vi "Periodic Tasks.vi"(8 "error in":errorcluster) -> ()   [LabVIEW 2019]
doc: "This VI runs in parallel to other tasks. It can contain as many user-defined periodic loops as you need. These can carry out PID or other sorts of timed response."
uses:
  <vilib>/Rock Robotics/WPI/ThirdParty/Phoenix-LabVIEW/Motor Controller/Controls/CTRE_Phoenix_MotorControl_ControlMode.ctl
  <vilib>/Rock Robotics/WPI/Solenoid/WPI_SolenoidValue.ctl
  Ball Routine.ctl
  TurretMode.ctl
  LabVIEW_is_Under_Control.lib/Util/Toggle/Change Detect.vi
  LabVIEW_is_Under_Control.lib/Util/Toggle/Change Detect Boolean.vi
  MotorsGlobal.vi
  <vilib>/Rock Robotics/WPI/Solenoid/WPI_SolenoidSetEnum.vi
  <vilib>/Rock Robotics/Network Tables/NT Read Number.vi
  JoysticksGlobal.vi
  <vilib>/Rock Robotics/WPI/Utilities/WPI_GetSetVariantRefNum.vi
  <vilib>/Rock Robotics/Network Tables/NT Write Number.vi
panel:
  out "Encoder Out":dbl
  in  "PIDs Tab":T1(tab)
  out "Current":dbl
  out "Motor Temperature":u8
  out "Current 2":dbl
  out "Motor Temperature 2":u8
  out "Current 3":dbl
  out "Motor Temperature 3":u8
  out "Current 4":dbl
  out "Motor Temperature 4":u8
  out "LimelightX":dbl
  out "Turret PID":cluster{"Setpoint":dbl, "Process variable":dbl}(graph)
  in  "Camera Angle":dbl=7.0
  out "Distancia do Goal":dbl
  in  "Inner Goal Height":dbl=2.49
  in  "Camera Height":dbl=0.185
  in  "Minimum command":dbl=0.031
  out "Turret Out":dbl
  in  "TAGains":T2={"proportional gain (Kc)"=1.0, "integral time (Ti, min)"=0.01, "derivative time (Td, min)"=0.0} {"derivative time (Td, min)" format="%.3f"; "integral time (Ti, min)" format="%.3f"; "proportional gain (Kc)" format="%.3f"}
  in  "TADisable Range":dbl
  in  "TAIntegral Range":dbl=10000.0
  in  "TASetpoint":dbl
  in  "TARange":cluster{"output high":dbl, "output low":dbl}={"output high"=0.6, "output low"=-0.6} {"output low" format="%.2f"; "output high" format="%.2f"}
  in  "kF":dbl=0.031
  out "Shooter PID":cluster{"Setpoint":dbl, "Process variable":dbl}(graph)
  in  "EnableFWPID":bool
  out "Variable":dbl
  in  "FWGains":T2={"proportional gain (Kc)"=1.0, "integral time (Ti, min)"=0.01, "derivative time (Td, min)"=0.0} {"derivative time (Td, min)" format="%.3f"; "integral time (Ti, min)" format="%.3f"; "proportional gain (Kc)" format="%.3f"}
  in  "FWRange":cluster{"output high":dbl, "output low":dbl}={"output high"=0.6, "output low"=-0.6} {"output low" format="%.2f"; "output high" format="%.2f"}
  in  "FWIntegral Range":dbl=10000.0
  in  "FWSetpoint":dbl
  in  "FWDisable Range":dbl
  # "System Tester"
  # "ID-1"
  # "ID-3"
  # "ID-2"
  # "ID-4"
  # "Distance Meter"
  # "All in cm"
  # "Turret Angle PID"
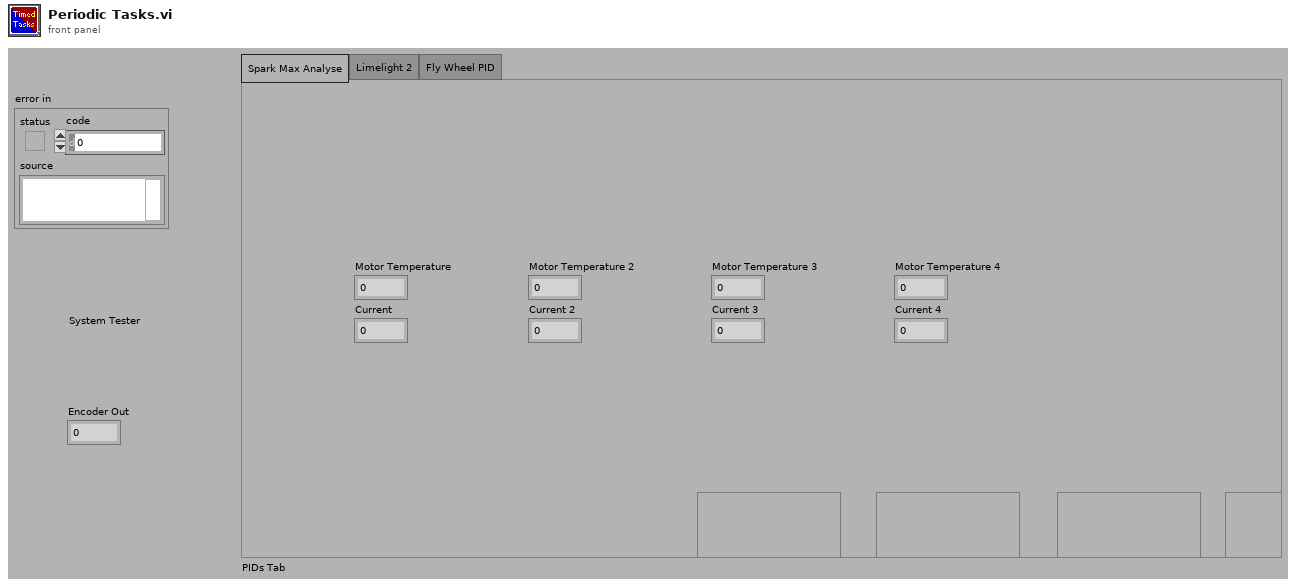
[diagram p1: front panel]
types:
  T1 = enum32{"Spark Max Analyse", "Limelight 2", "Fly Wheel PID"}
  T2 = cluster{"proportional gain (Kc)":dbl, "integral time (Ti, min)":dbl, "derivative time (Td, min)":dbl}
  T3 = typedef "WPI_SwitchDevRef.ctl" = cluster{"DevStatus":errorcluster, "DIO Channel":T4, "CntIndex":T5, "Normally Closed":bool}
  T4 = typedef "FPGA_DIOChannel.ctl" = enum8{"DIO 0", "DIO 1", "DIO 2", "DIO 3", "DIO 4", "DIO 5", "DIO 6", "DIO 7", "DIO 8", "DIO 9", "DIO MXP 0", "DIO MXP 1", "DIO MXP 2", "DIO MXP 3", "DIO MXP 4", "DIO MXP 5", "DIO MXP 6", "DIO MXP 7", "DIO MXP 8", "DIO MXP 9", "DIO MXP 10", "DIO MXP 11", "DIO MXP 12", "DIO MXP 13", "DIO MXP 14", "DIO MXP 15", "SPI Port CS1", "SPI Port CS2", "SPI Port CS3", "SPI Port MISO", "SPI Port MOSI", "Invalid"}
  T5 = typedef "FPGA_CounterCtrSystemIndex.ctl" = enum8{"Ctr 0", "Ctr 1", "Ctr 2", "Ctr 3", "Ctr 4", "Ctr 5", "Ctr 6", "Ctr 7", "Invalid"}
  T6 = typedef "WPI_EncoderDevRef.ctl" = cluster{"DevStatus":errorcluster, "EncoderIndex":T7, "CounterIndex":T5, "DistancePerCount":dbl, "Decoding Type":T8}
  T7 = typedef "FPGA_EncoderIdx.ctl" = enum8{"Enc 0", "Enc 1", "Enc 2", "Enc 3", "Enc 4", "Enc 5", "Enc 6", "Enc 7", "Invalid"}
  T8 = typedef "WPI_EncoderType.ctl" = enum16{"1x", "2x", "4x"}
  T9 = typedef "WPI_MotorControlDeviceRef.ctl" = cluster{"DeviceStatus":errorcluster, "Type":T10, "PWM":cluster{"PWM Channel":T11, "DeadBand":T12}, "CAN":cluster{"Device Number":u8, "SetOutput VI Ref":variant, "GetOutput VI Ref":variant, "Enable VI Ref":variant, "Disable VI Ref":variant, "Data":variant}, "Invert":bool, "DIO PWM":cluster{"PWM \"Enable\" Channel":T11, "DIOChannel":T4, "PWM Rate":dbl}}
  T10 = typedef "WPI_MotorControlType.ctl" = enum16{"PWM", "CAN", "DIO PWM"}
  T11 = typedef "FPGA_DIOPWMChannel.ctl" = enum8{"PWM 0", "PWM 1", "PWM 2", "PWM 3", "PWM 4", "PWM 5", "PWM 6", "PWM 7", "PWM 8", "PWM 9", "PWM MXP 0", "PWM MXP 1", "PWM MXP 2", "PWM MXP 3", "PWM MXP 4", "PWM MXP 5", "PWM MXP 6", "PWM MXP 7", "PWM MXP 8", "PWM MXP 9", "Invalid"}
  T12 = typedef "WPI_PWMDeadband.ctl" = cluster{"Name":string, "maxPositivePwm":i32, "minPositivePwm":i32, "centerPwm":i32, "maxNegativePwm":i32, "minNegativePwm":i32, "angularRange":u16}
  T13 = typedef "WPI_SolenoidDevRef.ctl" = cluster{"DevStatus":errorcluster, "Pneumatics Control Module":u8, "Forward Solenoid Channel":T14, "Reverse Solenoid Channel":T14}
  T14 = typedef "WPI_SolenoidChannel.ctl" = enum8{"Solenoid 0", "Solenoid 1", "Solenoid 2", "Solenoid 3", "Solenoid 4", "Solenoid 5", "Solenoid 6", "Solenoid 7", "Invalid"}
  T15 = typedef "WPI_SolenoidValue.ctl" = enum16{"Off", "On", "Forward", "Reverse"}
  T16 = typedef "CTRE_Phoenix_MotorControl_ControlMode.ctl" = u16
  T17 = typedef "WPI_RobotDriveDevRef.ctl" = cluster{"DevStatus":errorcluster, "Motors[]":T9[], "Square Inputs":bool, "Max Output":dbl}
  T18 = cluster{"Motors[][0]":T9, "Motors[][1]":T9, "Motors[][2]":T9, "Motors[][3]":T9, "Motors[][4]":T9, "Motors[][5]":T9, "Motors[][6]":T9, "Motors[][7]":T9, "Motors[][8]":T9}
  T19 = typedef "Ball Routine.ctl" = enum16{"Standart", "Get Power Cells", "Reset Intake", "Prepare Shooter", "Shoot!"}
  T20 = typedef "TurretMode.ctl" = enum16{"Static", "Manual", "Automatic"}
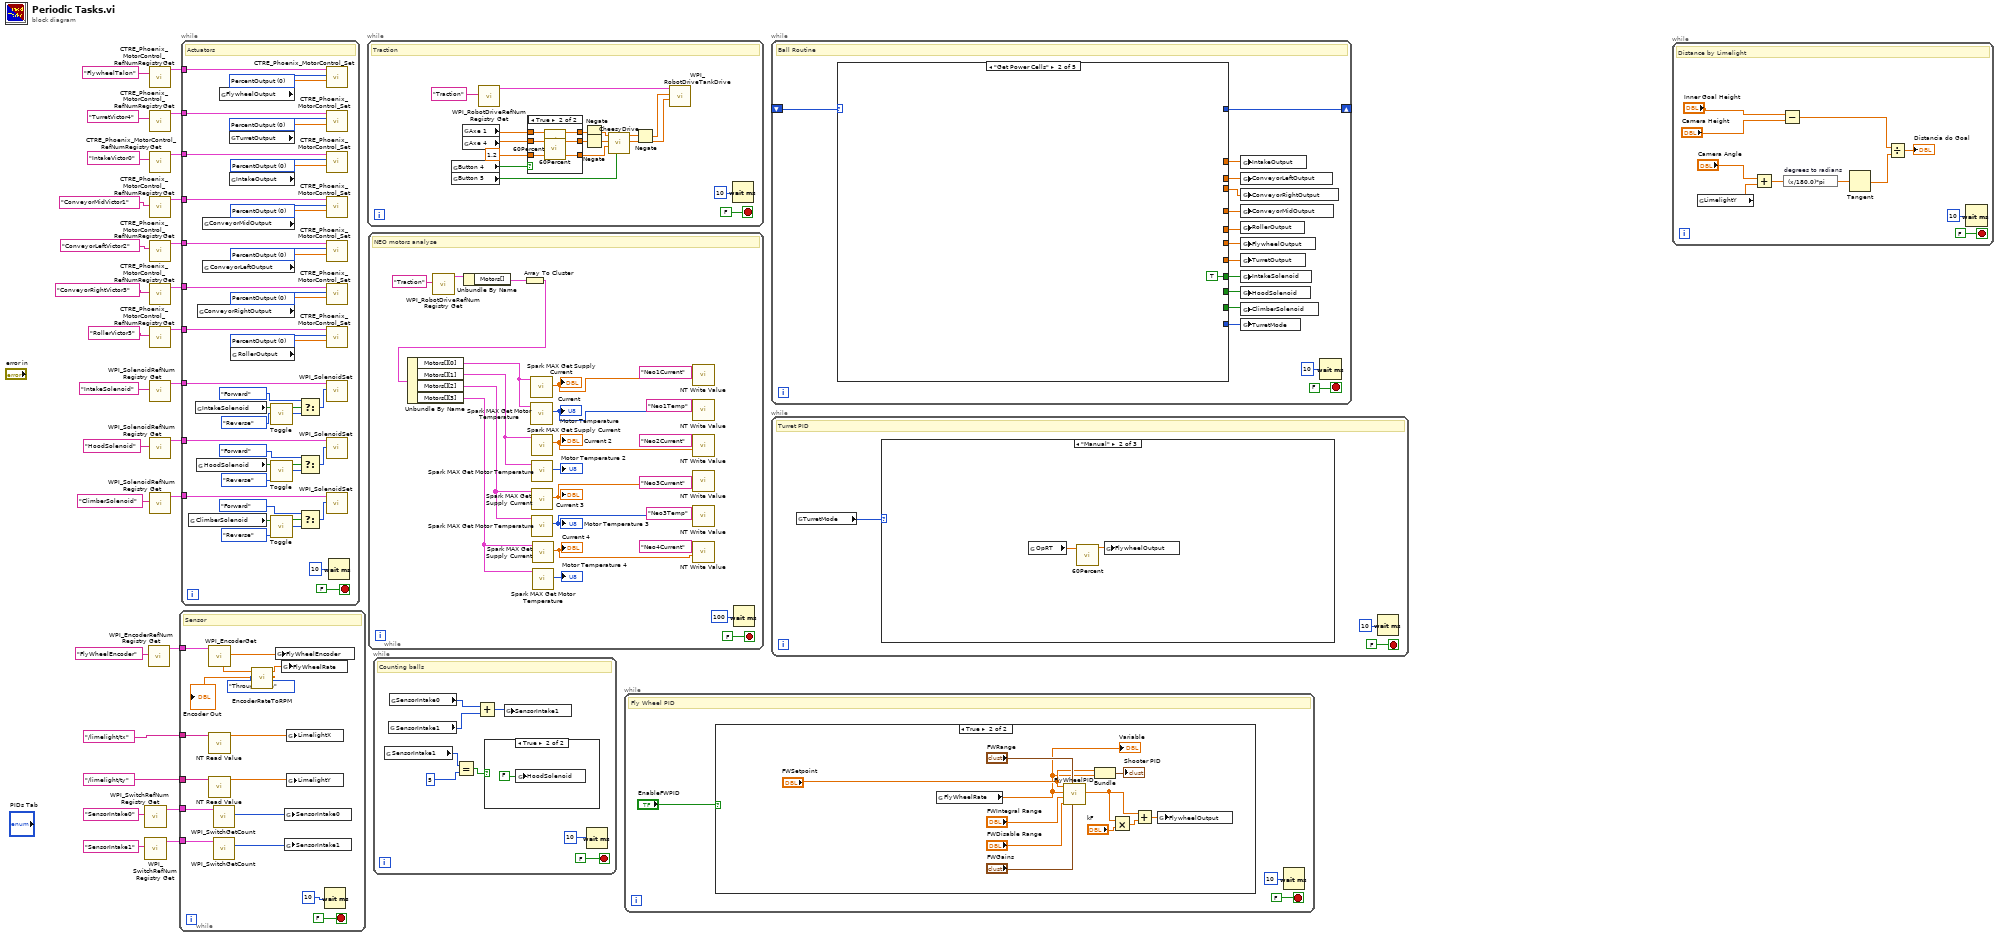
[diagram p0: block diagram]
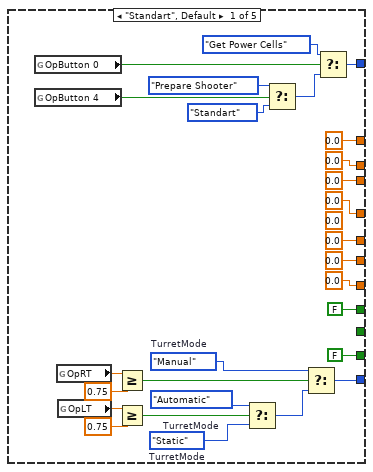
[diagram p3: hidden frame]
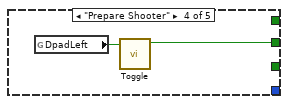
[diagram p5: hidden frame]
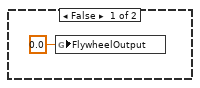
[diagram p7: hidden frame]
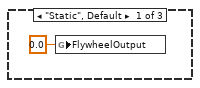
[diagram p8: hidden frame]
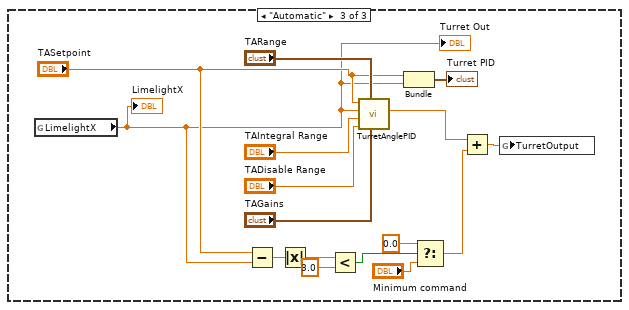
[diagram p9: hidden frame]
diagram:
  n1 = call <vilib>:"WPI_SwitchRefNum Registry Get.vi"("refnum name"="SensorIntake0") -> ("SwitchDevRef"=w3:T3)  [unwired: 9 in, 1 out]
  n2 = call <vilib>:"WPI_SwitchRefNum Registry Get.vi"("refnum name"="SensorIntake1") -> ("SwitchDevRef"=w4:T3)  [unwired: 9 in, 1 out]
  n3 = call <vilib>:"WPI_EncoderRefNum Registry Get.vi"("refnum name"="FlyWheelEncoder") -> ("EncoderDevRef"=w28:T6)  [unwired: 9 in, 1 out]
  n4 = call <vilib>:"CTRE_Phoenix_MotorControl_RefNumRegistryGet.vi"("refnum name"="FlywheelTalon") -> ("PhoenixMotorControlDevRef"=w23:T9)  [unwired: 9 in, 1 out]
  n5 = call <vilib>:"CTRE_Phoenix_MotorControl_RefNumRegistryGet.vi"("refnum name"="TurretVictor4") -> ("PhoenixMotorControlDevRef"=w22:T9)  [unwired: 9 in, 1 out]
  n6 = call <vilib>:"CTRE_Phoenix_MotorControl_RefNumRegistryGet.vi"("refnum name"="IntakeVictor0") -> ("PhoenixMotorControlDevRef"=w20:T9)  [unwired: 9 in, 1 out]
  n7 = call <vilib>:"CTRE_Phoenix_MotorControl_RefNumRegistryGet.vi"("refnum name"="ConveyorMidVictor1") -> ("PhoenixMotorControlDevRef"=w19:T9)  [unwired: 9 in, 1 out]
  n8 = call <vilib>:"CTRE_Phoenix_MotorControl_RefNumRegistryGet.vi"("refnum name"="ConveyorLeftVictor2") -> ("PhoenixMotorControlDevRef"=w18:T9)  [unwired: 9 in, 1 out]
  n9 = call <vilib>:"CTRE_Phoenix_MotorControl_RefNumRegistryGet.vi"("refnum name"="ConveyorRightVictor3") -> ("PhoenixMotorControlDevRef"=w17:T9)  [unwired: 9 in, 1 out]
  n10 = call <vilib>:"CTRE_Phoenix_MotorControl_RefNumRegistryGet.vi"("refnum name"="RollerVictor5") -> ("PhoenixMotorControlDevRef"=w5:T9)  [unwired: 9 in, 1 out]
  n11 = call <vilib>:"WPI_SolenoidRefNum Registry Get.vi"("refnum name"="IntakeSolenoid") -> ("SolenoidDevRef"=w12:T13)  [unwired: 9 in, 1 out]
  n12 = call <vilib>:"WPI_SolenoidRefNum Registry Get.vi"("refnum name"="HoodSolenoid") -> ("SolenoidDevRef"=w9:T13)  [unwired: 9 in, 1 out]
  n13 = call <vilib>:"WPI_SolenoidRefNum Registry Get.vi"("refnum name"="ClimberSolenoid") -> ("SolenoidDevRef"=w8:T13)  [unwired: 9 in, 1 out]
  n14 = while {
    tunnel: w28 -> [w42]
    tunnel: "/limelight/tx" ("Name") -> [w36]
    tunnel: "/limelight/ty" ("Name") -> [w33]
    tunnel: w4 -> [w31]
    tunnel: w3 -> [w32]
    stop <- FALSE stop-if-true
    # "Sensor"
    n15 = call <vilib>:"WPI_EncoderGet.vi"("EncoderDevRef"=w42) -> ("Distance"=w40:dbl, "Rate"=w39:dbl)  [unwired: 5 in, 4 out]
    n16 = call-poly <vilib>:"NT Read Value.vi"("Name"=w36) -> ("Numeric"=w35:dbl)  [unwired: 9 in, 1 out]
    n17 = call-poly <vilib>:"NT Read Value.vi"("Name"=w33) -> ("Numeric"=w34:dbl)  [unwired: 9 in, 1 out]
    n18 = call <vilib>:"WPI_SwitchGetCount.vi"("SwitchDevRef"=w32) -> ("Switch Pressed Count"=w30:i32)  [unwired: 8 in, 2 out]
    n19 = call <vilib>:"WPI_SwitchGetCount.vi"("SwitchDevRef"=w31) -> ("Switch Pressed Count"=w29:i32)  [unwired: 8 in, 2 out]
    n20 = call "EncoderRateToRPM.vi"("Enum"=enum16{"Through Bore", "Mag"}."Through Bore", "EncoderRate"=w39) -> ("RPM"=→"Encoder Out":dbl, "RPS"=w38:dbl)  [unwired: 8 in]
    n21 = global write "MotorsGlobal.vi" "FlyWheelEncoder"(w40) -> ()
    n22 = global write "MotorsGlobal.vi" "FlyWheelRate"(w38) -> ()
    n23 = global write "MotorsGlobal.vi" "SensorIntake0"(w30) -> ()
    n24 = global write "MotorsGlobal.vi" "SensorIntake1"(w29) -> ()
    n25 = global write "MotorsGlobal.vi" "LimelightX"(w35) -> ()
    n26 = global write "MotorsGlobal.vi" "LimelightY"(w34) -> ()
    n27 = Wait (ms)(milliseconds to wait=u32 10) -> ()  [unwired: 1 out]
  }
  n28 = while {
    tunnel: w23 -> [w82]
    tunnel: w22 -> [w81]
    tunnel: w20 -> [w77]
    tunnel: w19 -> [w76]
    tunnel: w18 -> [w75]
    tunnel: w17 -> [w74]
    tunnel: w12 -> [w65]
    tunnel: w9 -> [w54]
    tunnel: w8 -> [w53]
    tunnel: w5 -> [w45]
    stop <- FALSE stop-if-true
    w46 = T16 0 items=["PercentOutput"=0, "Position"=1, "Velocity"=2, "Current"=3, "Follower"=5, "MotionProfile"=6, "MotionMagic"=7, "MotionProfileArc"=10, "Disabled"=15] ("Control Mode")
    w67 = T16 0 items=["PercentOutput"=0, "Position"=1, "Velocity"=2, "Current"=3, "Follower"=5, "MotionProfile"=6, "MotionMagic"=7, "MotionProfileArc"=10, "Disabled"=15] ("Control Mode")
    w69 = T16 0 items=["PercentOutput"=0, "Position"=1, "Velocity"=2, "Current"=3, "Follower"=5, "MotionProfile"=6, "MotionMagic"=7, "MotionProfileArc"=10, "Disabled"=15] ("Control Mode")
    w71 = T16 0 items=["PercentOutput"=0, "Position"=1, "Velocity"=2, "Current"=3, "Follower"=5, "MotionProfile"=6, "MotionMagic"=7, "MotionProfileArc"=10, "Disabled"=15] ("Control Mode")
    w73 = T16 0 items=["PercentOutput"=0, "Position"=1, "Velocity"=2, "Current"=3, "Follower"=5, "MotionProfile"=6, "MotionMagic"=7, "MotionProfileArc"=10, "Disabled"=15] ("Control Mode")
    w79 = T16 0 items=["PercentOutput"=0, "Position"=1, "Velocity"=2, "Current"=3, "Follower"=5, "MotionProfile"=6, "MotionMagic"=7, "MotionProfileArc"=10, "Disabled"=15] ("Control Mode")
    w83 = T16 0 items=["PercentOutput"=0, "Position"=1, "Velocity"=2, "Current"=3, "Follower"=5, "MotionProfile"=6, "MotionMagic"=7, "MotionProfileArc"=10, "Disabled"=15] ("Control Mode")
    # "Actuators"
    n29 = global read "MotorsGlobal.vi" "ClimberSolenoid"() -> (w49:bool)
    n30 = global read "MotorsGlobal.vi" "IntakeSolenoid"() -> (w61:bool)
    n31 = global read "MotorsGlobal.vi" "HoodSolenoid"() -> (w58:bool)
    n32 = global read "MotorsGlobal.vi" "ConveyorRightOutput"() -> (w66:dbl)
    n33 = global read "MotorsGlobal.vi" "ConveyorMidOutput"() -> (w70:dbl)
    n34 = global read "MotorsGlobal.vi" "ConveyorLeftOutput"() -> (w68:dbl)
    n35 = global read "MotorsGlobal.vi" "FlywheelOutput"() -> (w80:dbl)
    n36 = global read "MotorsGlobal.vi" "TurretOutput"() -> (w78:dbl)
    n37 = global read "MotorsGlobal.vi" "IntakeOutput"() -> (w72:dbl)
    n38 = global read "MotorsGlobal.vi" "RollerOutput"() -> (w47:dbl)
    n39 = call "Toggle.vi"("In"=w61) -> ("Toggled"=w60:bool)  [unwired: 10 in]
    n40 = call "Toggle.vi"("In"=w58) -> ("Toggled"=w59:bool)  [unwired: 10 in]
    n41 = call "Toggle.vi"("In"=w49) -> ("Toggled"=w48:bool)  [unwired: 10 in]
    n42 = Select(t=WPI_SolenoidValue."Forward" ("Value"), s=w60, f=WPI_SolenoidValue."Reverse" ("Value")) -> (s? t:f=w63:T15)
    n43 = Select(t=WPI_SolenoidValue."Forward" ("Value"), s=w59, f=WPI_SolenoidValue."Reverse" ("Value")) -> (s? t:f=w56:T15)
    n44 = Select(t=WPI_SolenoidValue."Forward" ("Value"), s=w48, f=WPI_SolenoidValue."Reverse" ("Value")) -> (s? t:f=w51:T15)
    n45 = call <vilib>:"CTRE_Phoenix_MotorControl_Set.vi"("Output"=w80, "Control Mode"=w83, "PhoenixMotorControlDevRef"=w82) -> ()  [unwired: 7 in, 2 out]
    n46 = call <vilib>:"CTRE_Phoenix_MotorControl_Set.vi"("Output"=w78, "Control Mode"=w79, "PhoenixMotorControlDevRef"=w81) -> ()  [unwired: 7 in, 2 out]
    n47 = call <vilib>:"CTRE_Phoenix_MotorControl_Set.vi"("Output"=w72, "Control Mode"=w73, "PhoenixMotorControlDevRef"=w77) -> ()  [unwired: 7 in, 2 out]
    n48 = call <vilib>:"CTRE_Phoenix_MotorControl_Set.vi"("Output"=w70, "Control Mode"=w71, "PhoenixMotorControlDevRef"=w76) -> ()  [unwired: 7 in, 2 out]
    n49 = call <vilib>:"CTRE_Phoenix_MotorControl_Set.vi"("Output"=w68, "Control Mode"=w69, "PhoenixMotorControlDevRef"=w75) -> ()  [unwired: 7 in, 2 out]
    n50 = call <vilib>:"CTRE_Phoenix_MotorControl_Set.vi"("Output"=w66, "Control Mode"=w67, "PhoenixMotorControlDevRef"=w74) -> ()  [unwired: 7 in, 2 out]
    n51 = call <vilib>:"CTRE_Phoenix_MotorControl_Set.vi"("Output"=w47, "Control Mode"=w46, "PhoenixMotorControlDevRef"=w45) -> ()  [unwired: 7 in, 2 out]
    n52 = call-poly <vilib>:"WPI_SolenoidSet.vi"("Value"=w63, "SolenoidDevRef"=w65) -> ()  [unwired: 8 in, 2 out]
    n53 = call-poly <vilib>:"WPI_SolenoidSet.vi"("Value"=w56, "SolenoidDevRef"=w54) -> ()  [unwired: 8 in, 2 out]
    n54 = call-poly <vilib>:"WPI_SolenoidSet.vi"("Value"=w51, "SolenoidDevRef"=w53) -> ()  [unwired: 8 in, 2 out]
    n55 = Wait (ms)(milliseconds to wait=u32 10) -> ()  [unwired: 1 out]
  }
  n56 = while {
    stop <- FALSE stop-if-true
    # "Traction"
    n57 = global read "JoysticksGlobal.vi" "Button 4"() -> (w87:bool)
    n58 = global read "JoysticksGlobal.vi" "Button 5"() -> (w86:bool)
    n59 = global read "JoysticksGlobal.vi" "Axe 1"() -> (w91:dbl)
    n60 = global read "JoysticksGlobal.vi" "Axe 4"() -> (w90:dbl)
    n61 = call <vilib>:"WPI_RobotDriveRefNum Registry Get.vi"("refnum name"="Traction") -> ("RobotDriveDevRef"=w100:T17)  [unwired: 9 in, 1 out]
    n62 = case shown="True" w87 {
      tunnel: [w104 w110] -> w98
      tunnel: [w105 w109] -> w96
      tunnel: w91 -> [w105 w107]
      tunnel: w90 -> [w104 w108]
      tunnel: [w103 w106] -> w89
      tunnel: 1.2 ("Sensitivty") -> [w103 w106]
      frame False {
      }
      frame True {
        n63 = call "60Percent.vi"("In"=w107) -> ("Out"=w109:dbl)  [unwired: 9 in]
        n64 = call "60Percent.vi"("In"=w108) -> ("Out"=w110:dbl)  [unwired: 9 in]
      }
    }
    n65 = Negate(x=w96) -> (-x=w93:dbl)
    n66 = Negate(x=w98) -> (-x=w92:dbl)
    n67 = call "CheesyDrive.vi"("Quickturn"=w86, "Sensitivty"=w89, "Wheel"=w92, "Throttle"=w93) -> ("Right PWM"=w94:dbl, "Left PWM"=w97:dbl)  [unwired: 6 in]
    n68 = Negate(x=w97) -> (-x=w95:dbl)
    n69 = call <vilib>:"WPI_RobotDriveTankDrive.vi"("Right axis value"=w94, "Left axis value"=w95, "RobotDriveDevRef"=w100) -> ()  [unwired: 6 in, 3 out]
    n70 = Wait (ms)(milliseconds to wait=u32 10) -> ()  [unwired: 1 out]
  }
  n71 = while {
    stop <- FALSE stop-if-true
    # "NEO motors analyse"
    n72 = call <vilib>:"WPI_RobotDriveRefNum Registry Get.vi"("refnum name"="Traction") -> ("RobotDriveDevRef"=w133:T17)  [unwired: 9 in, 1 out]
    n73 = Unbundle By Name(w133) -> ("Motors[]"=w132:T9[])
    n74 = Array To Cluster(array=w132) -> (cluster=w126:T18)
    n75 = Unbundle By Name(w126) -> ("Motors[][0]"=w131:T9, "Motors[][1]"=w125:T9, "Motors[][2]"=w124:T9, "Motors[][3]"=w123:T9)
    n76 = call <vilib>:"Spark MAX Get Supply Current.vi"("MotorControlDevRef in"=w131) -> ("Current"=w121:dbl)  [unwired: 7 in, 3 out]
    "Current" <- w121
    n77 = call <vilib>:"Spark MAX Get Motor Temperature.vi"("MotorControlDevRef in"=w131) -> ("Motor Temperature"=w119:u8)  [unwired: 7 in, 3 out]
    "Motor Temperature" <- w119
    n78 = call <vilib>:"Spark MAX Get Supply Current.vi"("MotorControlDevRef in"=w125) -> ("Current"=w118:dbl)  [unwired: 7 in, 3 out]
    "Current 2" <- w118
    n79 = call <vilib>:"Spark MAX Get Motor Temperature.vi"("MotorControlDevRef in"=w125) -> ("Motor Temperature"=→"Motor Temperature 2":u8)  [unwired: 7 in, 3 out]
    n80 = call <vilib>:"Spark MAX Get Supply Current.vi"("MotorControlDevRef in"=w124) -> ("Current"=w117:dbl)  [unwired: 7 in, 3 out]
    "Current 3" <- w117
    n81 = call <vilib>:"Spark MAX Get Motor Temperature.vi"("MotorControlDevRef in"=w124) -> ("Motor Temperature"=w116:u8)  [unwired: 7 in, 3 out]
    "Motor Temperature 3" <- w116
    n82 = call <vilib>:"Spark MAX Get Supply Current.vi"("MotorControlDevRef in"=w123) -> ("Current"=w115:dbl)  [unwired: 7 in, 3 out]
    "Current 4" <- w115
    n83 = call <vilib>:"Spark MAX Get Motor Temperature.vi"("MotorControlDevRef in"=w123) -> ("Motor Temperature"=→"Motor Temperature 4":u8)  [unwired: 7 in, 3 out]
    n84 = call-poly <vilib>:"NT Write Value.vi"("Numeric"=w121, "Name"="Neo1Current") -> ()  [unwired: 9 in, 1 out]
    n85 = call-poly <vilib>:"NT Write Value.vi"("Numeric"=w119, "Name"="Neo1Temp") -> ()  [unwired: 9 in, 1 out]
    n86 = call-poly <vilib>:"NT Write Value.vi"("Numeric"=w118, "Name"="Neo2Current") -> ()  [unwired: 9 in, 1 out]
    n87 = call-poly <vilib>:"NT Write Value.vi"("Numeric"=w117, "Name"="Neo3Current") -> ()  [unwired: 9 in, 1 out]
    n88 = call-poly <vilib>:"NT Write Value.vi"("Numeric"=w116, "Name"="Neo3Temp") -> ()  [unwired: 9 in, 1 out]
    n89 = call-poly <vilib>:"NT Write Value.vi"("Numeric"=w115, "Name"="Neo4Current") -> ()  [unwired: 9 in, 1 out]
    n90 = Wait (ms)(milliseconds to wait=u32 100) -> ()  [unwired: 1 out]
  }
  n91 = while {
    stop <- FALSE stop-if-true
    # "Counting balls"
    n92 = global read "MotorsGlobal.vi" "SensorIntake1"() -> (w136:i32)
    n93 = global read "MotorsGlobal.vi" "SensorIntake1"() -> (w139:i32)
    n94 = global read "MotorsGlobal.vi" "SensorIntake0"() -> (w140:i32)
    n95 = Equal?(x=w136, y=5) -> (x = y?=w137:bool)
    n96 = Add(x=w140, y=w139) -> (x+y=w138:i32)
    n97 = case shown="True" w137 {
      frame False {
      }
      frame True {
        n98 = global write "MotorsGlobal.vi" "HoodSolenoid"(FALSE ("HoodSolenoid")) -> ()
      }
    }
    n99 = global write "MotorsGlobal.vi" "SensorIntake1"(w138) -> ()
    n100 = Wait (ms)(milliseconds to wait=u32 10) -> ()  [unwired: 1 out]
  }
  n101 = while {
    stop <- FALSE stop-if-true
    # "Fly Wheel PID"
    n102 = case shown="True" "EnableFWPID" {
      frame False {
        n103 = global write "MotorsGlobal.vi" "FlywheelOutput"(0.0 ("FlywheelOutput")) -> ()
      }
      frame True {
        n104 = global read "MotorsGlobal.vi" "FlyWheelRate"() -> (w153:dbl)
        "Variable" <- w153
        n105 = call "FlyWheelPID.vi"("FWGains"="FWGains", "FWRange"="FWRange", "FWDisable Range"="FWDisable Range", "FWIntegral Range"="FWIntegral Range", "FWProcess variable"=w153, "FWSetpoint"="FWSetpoint") -> ("FWoutput"=w149:dbl)  [unwired: 4 in]
        n106 = Bundle("FWSetpoint"="FWSetpoint", "FlyWheelRate"=w153) -> (→"Shooter PID":cluster{"FWSetpoint":dbl, "FlyWheelRate":dbl})  [unwired: 1 in]
        n107 = Multiply(x=w149, y="kF") -> (x*y=w150:dbl)
        n108 = Add(x=w149, y=w150) -> (x+y=w148:dbl)
        n109 = global write "MotorsGlobal.vi" "FlywheelOutput"(w148) -> ()
      }
    }
    n110 = Wait (ms)(milliseconds to wait=u32 10) -> ()  [unwired: 1 out]
  }
  n111 = while {
    shift-right: [w170] -> _
    shift-left: _ -> [w171]
    stop <- FALSE stop-if-true
    # "Ball Routine"
    n112 = case shown="\"Get Power Cells\"" w171 {
      tunnel: [w200 _ _ _ _] -> w170
      tunnel: [0.0 _ _ _ _] -> w169
      tunnel: [0.0 _ _ _ _] -> w168
      tunnel: [0.0 _ _ _ _] -> w167
      tunnel: [0.0 _ _ _ _] -> w166
      tunnel: [0.0 _ _ _ _] -> w165
      tunnel: [0.0 _ _ _ _] -> w164
      tunnel: [0.0 _ _ _ _] -> w163
      tunnel: [FALSE ("IntakeSolenoid") TRUE ("IntakeSolenoid") _ _ _] -> w162
      tunnel: [FALSE ("IntakeSolenoid") _ _ _ _] -> w161
      tunnel: [_ _ _ w202 _] -> w160
      tunnel: [w184 _ _ _ _] -> w159
      frame "Standart", Default {
        w174 = TurretMode."Manual"  # TurretMode
        w175 = TurretMode."Automatic"  # TurretMode
        w182 = TurretMode."Static"  # TurretMode
        (unwired) 0.0
        n113 = global read "JoysticksGlobal.vi" "OpButton 0"() -> (w186:bool)
        n114 = global read "JoysticksGlobal.vi" "OpButton 4"() -> (w187:bool)
        n115 = global read "JoysticksGlobal.vi" "OpRT"() -> (w178:dbl)
        n116 = global read "JoysticksGlobal.vi" "OpLT"() -> (w181:dbl)
        n117 = Greater Or Equal?(x=w178, y=0.75) -> (x >= y?=w176:bool)
        n118 = Greater Or Equal?(x=w181, y=0.75) -> (x >= y?=w177:bool)
        n119 = Select(t=w175, s=w177, f=w182) -> (s? t:f=w183:T20)
        n120 = Select(t=Ball_Routine."Prepare Shooter", s=w187, f=Ball_Routine."Standart") -> (s? t:f=w190:T19)
        n121 = Select(t=w174, s=w176, f=w183) -> (s? t:f=w184:T20)
        n122 = Select(t=Ball_Routine."Get Power Cells", s=w186, f=w190) -> (s? t:f=w200:T19)
      }
      frame "Get Power Cells" {
      }
      frame "Reset Intake" {
      }
      frame "Prepare Shooter" {
        n123 = global read "JoysticksGlobal.vi" "DpadLeft"() -> (w203:bool)
        n124 = call "Toggle.vi"("In"=w203) -> ("Toggled"=w202:bool)  [unwired: 10 in]
      }
      frame "Shoot!" {
      }
    }
    n125 = global write "MotorsGlobal.vi" "IntakeOutput"(w169) -> ()
    n126 = global write "MotorsGlobal.vi" "ConveyorLeftOutput"(w165) -> ()
    n127 = global write "MotorsGlobal.vi" "ConveyorRightOutput"(w164) -> ()
    n128 = global write "MotorsGlobal.vi" "ConveyorMidOutput"(w163) -> ()
    n129 = global write "MotorsGlobal.vi" "RollerOutput"(w166) -> ()
    n130 = global write "MotorsGlobal.vi" "FlywheelOutput"(w167) -> ()
    n131 = global write "MotorsGlobal.vi" "TurretOutput"(w168) -> ()
    n132 = global write "MotorsGlobal.vi" "IntakeSolenoid"(w162) -> ()
    n133 = global write "MotorsGlobal.vi" "HoodSolenoid"(w160) -> ()
    n134 = global write "MotorsGlobal.vi" "ClimberSolenoid"(w161) -> ()
    n135 = global write "MotorsGlobal.vi" "TurretMode"(w159) -> ()
    n136 = Wait (ms)(milliseconds to wait=u32 10) -> ()  [unwired: 1 out]
  }
  n137 = while {
    stop <- FALSE stop-if-true
    # "Turret PID"
    n138 = global read "MotorsGlobal.vi" "TurretMode"() -> (w204:T20)
    n139 = case shown="\"Manual\"" w204 {
      frame "Static", Default {
        n140 = global write "MotorsGlobal.vi" "FlywheelOutput"(0.0 ("FlywheelOutput")) -> ()
      }
      frame "Manual" {
        n141 = global read "JoysticksGlobal.vi" "OpRT"() -> (w209:dbl)
        n142 = call "60Percent.vi"("In"=w209) -> ("Out"=w208:dbl)  [unwired: 9 in]
        n143 = global write "MotorsGlobal.vi" "FlywheelOutput"(w208) -> ()
      }
      frame "Automatic" {
        n144 = global read "MotorsGlobal.vi" "LimelightX"() -> (w217:dbl)
        "Turret Out" <- w217
        "LimelightX" <- w217
        n145 = Subtract(x="TASetpoint", y=w217) -> (x-y=w216:dbl)
        n146 = Absolute Value(x=w216) -> (abs(x)=w215:dbl)
        n147 = Less?(x=w215, y=3.0) -> (x < y?=w213:bool)
        n148 = call "TurretAnglePID.vi"("TAGains"="TAGains", "TARange"="TARange", "TADisable Range"="TADisable Range", "TAIntegral Range"="TAIntegral Range", "TAProcess variable"=w217, "TASetpoint"="TASetpoint") -> ("TAoutput"=w219:dbl)  [unwired: 5 in]
        n149 = Bundle("TASetpoint"="TASetpoint", "LimelightX"=w217) -> (→"Turret PID":cluster{"TASetpoint":dbl, "LimelightX":dbl})  [unwired: 1 in]
        n150 = Select(t=0.0, s=w213, f="Minimum command") -> (s? t:f=w210:dbl)
        n151 = Add(x=w219, y=w210) -> (x+y=w224:dbl)
        n152 = global write "MotorsGlobal.vi" "TurretOutput"(w224) -> ()
      }
    }
    n153 = Wait (ms)(milliseconds to wait=u32 10) -> ()  [unwired: 1 out]
  }
  n154 = while {
    stop <- FALSE stop-if-true
    # "Distance by Limelight"
    n155 = global read "MotorsGlobal.vi" "LimelightY"() -> (w226:dbl)
    n156 = Add(x="Camera Angle", y=w226) -> (x+y=w228:dbl)
    n157 = Subtract(x="Inner Goal Height", y="Camera Height") -> (x-y=w235:dbl)
    n158 = expression code="(x/180.0)*pi" "degrees to radians"(w228) -> (w229:dbl)
    n159 = Tangent(1:w229) -> (0:w236:dbl)
    n160 = Divide(x=w235, y=w236) -> (x/y=→"Distancia do Goal":dbl)
    n161 = Wait (ms)(milliseconds to wait=u32 10) -> ()  [unwired: 1 out]
  }
